vi "791_sweep_count.vi"() -> ()   [LabVIEW 2009]
uses:
  <vilib>/DAQmx/configure/timing.llb/DAQmx Timing (Implicit).vi
  <vilib>/DAQmx/create/channels.llb/DAQmx Create Channel (CO-Pulse Generation-Frequency).vi
  <vilib>/DAQmx/configure/timing.llb/DAQmx Timing (Sample Clock).vi
  <vilib>/DAQmx/create/channels.llb/DAQmx Create Channel (CI-Count Edges).vi
  <vilib>/DAQmx/create/channels.llb/DAQmx Create Channel (AI-Voltage-Basic).vi
  <vilib>/DAQmx/read.llb/DAQmx Read (Counter U32 1Chan 1Samp).vi
  <vilib>/DAQmx/read.llb/DAQmx Read (Analog DBL 1Chan 1Samp).vi
  Program Files/National Instruments/LabVIEW 2009/resource/objmgr/daqmx.rc
panel:
  in  "Samples  in stack":i32=100 min=1 step=1
  out "array":dbl[](graph)
  out "Voltage":dbl(graph)
  in  "stop":bool
  in  "Sample Time":dbl=0.02 step=0.0001
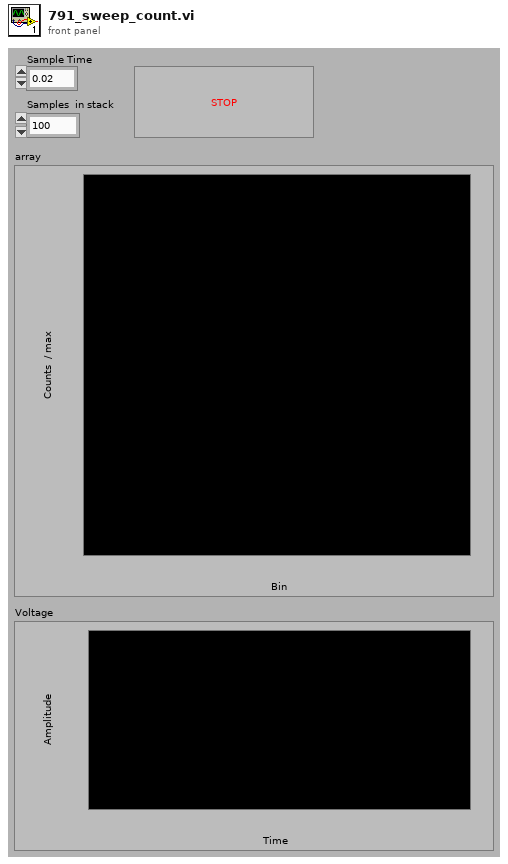
[diagram p1: front panel]
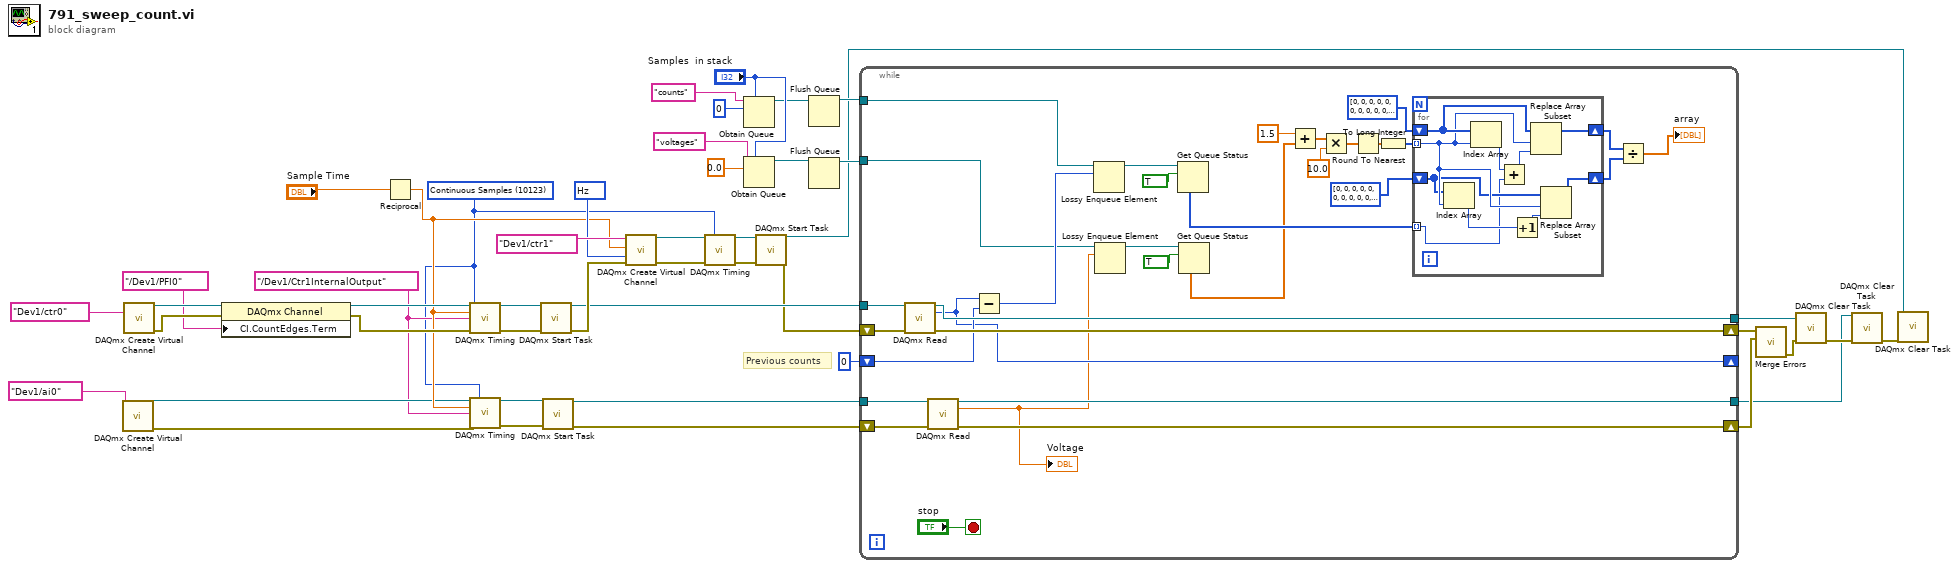
[diagram p0: block diagram]
diagram:
  w25 = tag "/Dev1/Ctr1InternalOutput" ("source")
  w42 = 10373 items=["Hz"=10373] ("units")
  w24 = 10123 items=["Finite Samples"=10178, "Continuous Samples"=10123, "Hardware Timed Single Point"=12522] ("sample mode")
  # "Previous counts"
  n1 = call-poly <vilib>:"DAQmx Create Virtual Channel.vi"("physical channels"=tag "Dev1/ai0") -> ("task out"=w27:refnum<k21>, "error out"=w26:errorcluster)  [unwired: 13 in]
  n2 = call-poly <vilib>:"DAQmx Create Virtual Channel.vi"("counter"=tag "Dev1/ctr0") -> ("task out"=w34:refnum<k21>, "error out"=w33:errorcluster)  [unwired: 13 in]
  n3 = property class="DAQmx Channel"(reference=w34, error in=w33, "CI.CountEdges.Term"=tag "/Dev1/PFI0") -> (reference out=w36:refnum<k21>, error out=w35:errorcluster)
  n4 = Reciprocal(x="Sample Time") -> (1/x=w28:dbl)
  n5 = call-poly <vilib>:"DAQmx Timing.vi"("task/channels in"=w36, "sample mode"=w24, "rate"=w28, "source"=w25, "error in"=w35) -> ("task out"=w45:refnum<k21>, "error out"=w44:errorcluster)  [unwired: 9 in]
  n6 = call-poly <vilib>:"DAQmx Timing.vi"("task/channels in"=w27, "sample mode"=w24, "rate"=w28, "source"=w25, "error in"=w26) -> ("task out"=w23:refnum<k21>, "error out"=w22:errorcluster)  [unwired: 9 in]
  n7 = call <vilib>:"DAQmx Start Task.vi"("task/channels in"=w45, "error in"=w44) -> ("task out"=w30:refnum<k21>, "error out"=w37:errorcluster)  [unwired: 12 in]
  n8 = call <vilib>:"DAQmx Start Task.vi"("task/channels in"=w23, "error in"=w22) -> ("task out"=w21:refnum<k21>, "error out"=w20:errorcluster)  [unwired: 12 in]
  n9 = call-poly <vilib>:"DAQmx Create Virtual Channel.vi"("frequency"=w28, "counter"=tag "Dev1/ctr1", "units"=w42, "error in"=w37) -> ("task out"=w41:refnum<k21>, "error out"=w40:errorcluster)  [unwired: 10 in]
  n10 = call-poly <vilib>:"DAQmx Timing.vi"("task/channels in"=w41, "sample mode"=w24, "error in"=w40) -> ("task out"=w39:refnum<k21>, "error out"=w38:errorcluster)  [unwired: 11 in]
  n11 = Obtain Queue(max queue size (-1, unlimited)="Samples  in stack", name (unnamed)="counts", element data type=u32 0) -> (queue out=w11:refnum<queue>)  [unwired: 2 in, 2 out]
  n12 = Obtain Queue(max queue size (-1, unlimited)="Samples  in stack", name (unnamed)="voltages", element data type=0.0) -> (queue out=w9:refnum<queue>)  [unwired: 2 in, 2 out]
  n13 = call <vilib>:"DAQmx Start Task.vi"("task/channels in"=w39, "error in"=w38) -> ("task out"=w7:refnum<k21>, "error out"=w19:errorcluster)  [unwired: 12 in]
  n14 = Flush Queue(queue=w11) -> (queue out=w10:refnum<queue>)  [unwired: 1 in, 2 out]
  n15 = Flush Queue(queue=w9) -> (queue out=w8:refnum<queue>)  [unwired: 1 in, 2 out]
  n16 = while {
    tunnel: w30 -> [w77]
    tunnel: w21 -> [w76]
    tunnel: [w75] -> w1
    tunnel: [w74] -> w18
    shift-right: [w72] -> w5
    shift-left: w19 -> [w71]
    shift-right: [w70] -> w4
    shift-left: w20 -> [w73]
    shift-right: [w68] -> _
    shift-left: u32 0 ("data") -> [w69]
    tunnel: w10 -> [w54]
    tunnel: w8 -> [w49]
    stop <- "stop" stop-if-true
    n17 = call-poly <vilib>:"DAQmx Read.vi"("task/channels in"=w77, "error in"=w71) -> ("task out"=w74:refnum<k21>, "data"=w68:u32, "error out"=w72:errorcluster)  [unwired: 11 in]
    n18 = call-poly <vilib>:"DAQmx Read.vi"("task/channels in"=w76, "error in"=w73) -> ("task out"=w75:refnum<k21>, "data"=w47:dbl, "error out"=w70:errorcluster)  [unwired: 11 in]
    "Voltage" <- w47
    n19 = Subtract(x=w68, y=w69) -> (x-y=w53:u32)
    n20 = Lossy Enqueue Element(queue=w54, element=w53) -> (queue out=w56:refnum<queue>)  [unwired: 1 in, 3 out]
    n21 = Lossy Enqueue Element(queue=w49, element=w47) -> (queue out=w51:refnum<queue>)  [unwired: 1 in, 3 out]
    n22 = Get Queue Status(queue=w56, return elements? (F)=TRUE) -> (elements=w52:u32[])  [unwired: 1 in, 7 out]
    n23 = Get Queue Status(queue=w51, return elements? (F)=TRUE) -> (elements=w48:dbl[])  [unwired: 1 in, 7 out]
    n24 = Add(x=1.5, y=w48) -> (x+y=w67:dbl[])
    n25 = Multiply(x=w67, y=10.0) -> (x*y=w64:dbl[])
    n26 = Round To Nearest(number=w64) -> (nearest integer value=w63:dbl[])
    n27 = To Long Integer(number=w63) -> (32bit integer=w62:i32[])
    n28 = for {
      tunnel: w62 -> [w82] mode=indexing
      shift-right: [w85] -> w58
      shift-left: u32[] [0, 0, 0, 0, 0, 0, 0, 0, 0, 0, 0, 0, 0, 0, 0, 0, 0, 0, 0, 0, 0, 0, 0, 0, 0, 0, 0, 0, 0, 0, 0, 0, 0, 0, 0, 0, 0, 0, 0, 0, 0, 0, 0, 0, 0, 0, 0, 0, 0, 0, 0, 0, 0, 0, 0, 0, 0, 0, 0, 0, 0, 0, 0, 0, 0, 0, 0, 0, 0, 0, 0, 0, 0, 0, 0, 0, 0, 0, 0, 0, 0, 0, 0, 0, 0, 0, 0, 0, 0, 0, 0, 0, 0, 0, 0, 0, 0, 0, 0, 0, 0] ("array") -> [w87]
      shift-right: [w80] -> w59
      shift-left: u32[] [0, 0, 0, 0, 0, 0, 0, 0, 0, 0, 0, 0, 0, 0, 0, 0, 0, 0, 0, 0, 0, 0, 0, 0, 0, 0, 0, 0, 0, 0, 0, 0, 0, 0, 0, 0, 0, 0, 0, 0, 0, 0, 0, 0, 0, 0, 0, 0, 0, 0, 0, 0, 0, 0, 0, 0, 0, 0, 0, 0, 0, 0, 0, 0, 0, 0, 0, 0, 0, 0, 0, 0, 0, 0, 0, 0, 0, 0, 0, 0, 0, 0, 0, 0, 0, 0, 0, 0, 0, 0, 0, 0, 0, 0, 0, 0, 0, 0, 0, 0, 0] ("array") -> [w81]
      tunnel: w52 -> [w79] mode=indexing
      n29 = Index Array(array=w81, index=w82) -> (element=w84:u32)
      n30 = Index Array(array=w87, index=w82) -> (element=w88:u32)
      n31 = Add(x=w88, y=w79) -> (x+y=w86:u32)
      n32 = Increment(x=w84) -> (x+1=w83:u32)
      n33 = Replace Array Subset(array=w87, new element=w86, index=w82) -> (w85:u32[])
      n34 = Replace Array Subset(array=w81, new element=w83, index=w82) -> (w80:u32[])
    }
    n35 = Divide(x=w58, y=w59) -> (x/y=→"array":dbl[])
  }
  n36 = call <vilib>:"Merge Errors.vi"("error in 2 (no error)"=w4, "error in 1 (no error)"=w5) -> ("error out"=w6:errorcluster)  [unwired: 5 in]
  n37 = call <vilib>:"DAQmx Clear Task.vi"("task in"=w18, "error in"=w6) -> ("error out"=w3:errorcluster)  [unwired: 13 in]
  n38 = call <vilib>:"DAQmx Clear Task.vi"("task in"=w1, "error in"=w3) -> ("error out"=w2:errorcluster)  [unwired: 13 in]
  n39 = call <vilib>:"DAQmx Clear Task.vi"("task in"=w7, "error in"=w2) -> ()  [unwired: 13 in, 1 out]
